vi "Logger_Create.vi"(0 "reference in":refnum<class "Logger.lvclass">, 1 "Logger Queue":refnum<queue>, 2 "Output Directory":path, 3 "HPS17K Refs":refnum<class "HPS-17000.lvclass">[](array[class]), 5 "Error In":errorcluster, 6 "Log File Type":enum16{"TDMS", "CSV"}(ring)) -> (14 "reference out":refnum<class "Logger.lvclass">, 19 "Error Out":errorcluster)   [LabVIEW 2023, in "Logger.lvclass"]
uses:
  Logger.lvclass
  <vilib>/HPS-17000/MStream_grpc_CyclerMeasurement.ctl
  <instrlib>/HPS-17000/HPS-17000.lvclass
  Logger.lvclass/Logger.ctl
  <vilib>/HPS-17000/NI_BC_client.lvlib
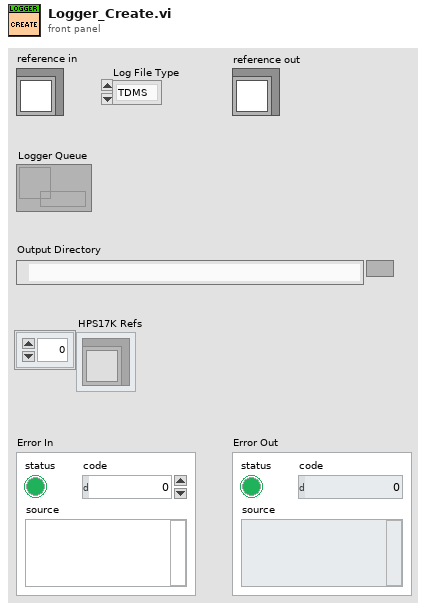
[diagram p1: front panel]
types:
  T1 = typedef "Logger.lvclass/ObjectAttributes.ctl" = cluster{"Output Directory":path, "Log File Type":enum16{"TDMS", "CSV"}, "Logger Queue":refnum<queue>, "HPS17K Refs":refnum<class "HPS-17000.lvclass">[]}
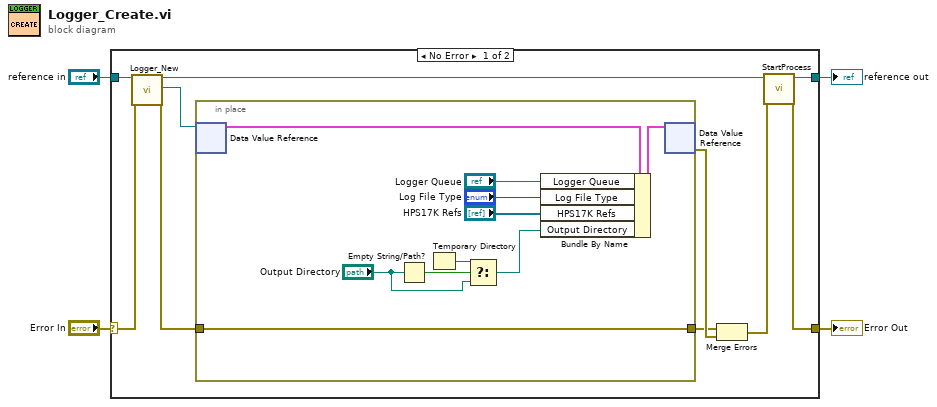
[diagram p0: block diagram]
diagram:
  n1 = case shown="No Error" "Error In" {
    selector: "Error In" -> [w13 w26]
    tunnel: [w5 w26] -> w3
    tunnel: "reference in" -> [w14 w25]
    tunnel: [w7 w25] -> w1
    frame No Error {
      n2 = call "Logger_New.vi"("reference in"=w14, "Error In"=w13) -> ("reference out"=w8:refnum<class "Logger.lvclass">, "DVRRefOut"=w11:refnum<data-value>, "Error Out"=w10:errorcluster)  [unwired: 14 in, 1 out]
      n3 = in-place {
        in-place-border: w10 -> [w22]
        in-place-border: [w22] -> w9
        n4 = in-place-dvr #1(w11) -> (w23:T1)  [unwired: 1 out]
        n5 = Empty String/Path?(string/path="Output Directory") -> (empty?=w18:bool)
        n6 = Temporary Directory() -> (w17:path)
        n7 = Select(t=w17, s=w18, f="Output Directory") -> (s? t:f=w15:path)
        n8 = Bundle By Name(cluster=w23, "Logger Queue"="Logger Queue", "Log File Type"="Log File Type", "HPS17K Refs"="HPS17K Refs", "Output Directory"=w15) -> (w24:T1)
        n9 = in-place-dvr #1(w24) -> (w12:errorcluster)  [unwired: 1 out]
      }
      n10 = Merge Errors(w9, w12) -> (w6:errorcluster)
      n11 = call "StartProcess.vi"("reference in"=w8, "Error In"=w6) -> ("reference out"=w7:refnum<class "Logger.lvclass">, "Error Out"=w5:errorcluster)  [unwired: 14 in, 2 out]
    }
    frame Error {
      # "VI-TechBaseTemplate_Simple_6x8x6"
    }
  }
  "Error Out" <- w3
  "reference out" <- w1
